vi "Init Test.vi"(10 "x":dbl, 11 "Cluster":T1) -> (3 "output cluster":T1)   [LabVIEW 2013]
uses:
  Control/SystemProcess.ctl
  Control/Buffer.vi
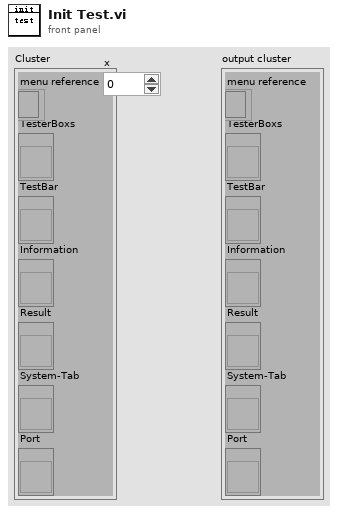
[diagram p1: front panel]
types:
  T1 = cluster{"menu reference":refnum<k9>, "TesterBoxs":refnum<vi>, "TestBar":refnum<vi>, "Information":refnum<vi>, "Result":refnum<vi>, "System-Tab":refnum<vi>, "Port":refnum<vi>}
  T2 = typedef "SystemProcess.ctl" = enum16{"Idle", "SystemInit", "SpecialEvent", "Barcode(SN)", "TestInitialize", "Test", "Stop", "SaveTestData", "Exit"}
  T3 = typedef "StatusInformation.ctl" = cluster{"FileName:":string, "Barcode(S/N):":string, "TestStep:":string, "TestTime:":string, "Station:":string, "Model:":string, "Line:":string, "Status:":string, "Series:":string, "Reserve:":string}
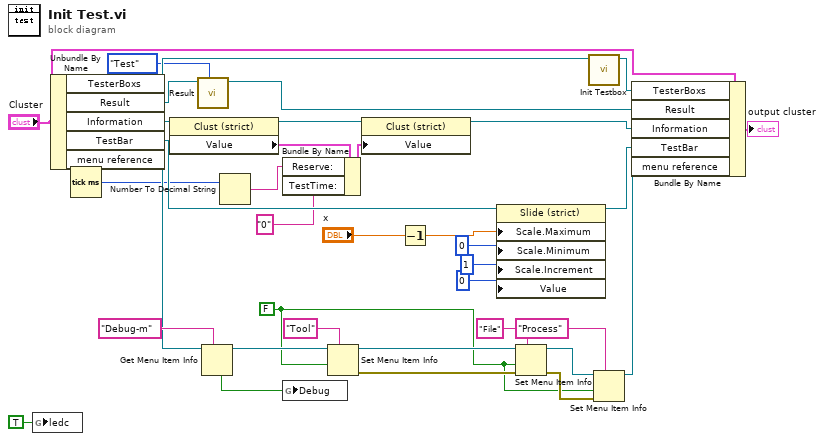
[diagram p0: block diagram]
diagram:
  w4 = FALSE ("enabled")
  n1 = global write "Buffer.vi" "ledc"(TRUE ("ledc")) -> ()
  n2 = Unbundle By Name("Cluster") -> ("TesterBoxs"=w31:refnum<vi>, "Result"=w28:refnum<vi>, "Information"=w30:refnum<vi>, "TestBar"=w33:refnum<vi>, "menu reference"=w3:refnum<k9>)
  n3 = Tick Count (ms)() -> (millisecond timer value=w1:u32)
  n4 = property class="Clust (strict)"(reference=w30) -> (reference out=w21:refnum<vi>, "Value"=w22:T3)  [unwired: 1 in, 1 out]
  n5 = call "Result.vi"("MainProcess"=SystemProcess."Test", "Result"=w28) -> ("Result"=w29:refnum<vi>)  [unwired: 9 in]
  n6 = Get Menu Item Info(7:"Debug-m" ("item tag"), 11:w3) -> (3:w17:refnum<k9>, 4:w25:bool)  [unwired: 1 in, 5 out]
  n7 = Number To Decimal String(number=w1) -> (decimal integer string=w18:string)  [unwired: 1 in]
  n8 = Bundle By Name(cluster=w22, "Reserve:"=w18, "TestTime:"="0") -> (w19:T3)
  n9 = global write "Buffer.vi" "Debug"(w25) -> ()
  n10 = Set Menu Item Info(7:"Tool" ("item tag"), 9:w4, 11:w17) -> (0:w14:errorcluster, 3:w15:refnum<k9>)  [unwired: 4 in]
  n11 = property class="Clust (strict)"(reference=w21, "Value"=w19) -> (reference out=w20:refnum<vi>)  [unwired: 1 in, 1 out]
  n12 = Decrement(x="x") -> (x-1=w23:dbl)
  n13 = property class="Slide (strict)"(reference=w33, "Scale.Maximum"=w23, "Scale.Minimum"=0 ("Data Entry Limits:Minimum"), "Scale.Increment"=1 ("Data Entry Limits:Increment"), "Value"=0) -> (reference out=w34:refnum<vi>)  [unwired: 1 in, 1 out]
  n14 = Set Menu Item Info(7:"File" ("item tag"), 8:w14, 9:w4, 11:w15) -> (0:w6:errorcluster, 3:w8:refnum<k9>)  [unwired: 3 in]
  n15 = call "Init Testbox.vi"("MulticolumnListbox in"=w31) -> ("MulticolumnListbox in"=w32:refnum<vi>)  [unwired: 10 in]
  n16 = Set Menu Item Info(7:"Process" ("item tag"), 8:w6, 9:w4, 11:w8) -> (3:w7:refnum<k9>)  [unwired: 3 in, 1 out]
  n17 = Bundle By Name(cluster="Cluster", "TesterBoxs"=w32, "Result"=w29, "Information"=w20, "TestBar"=w34, "menu reference"=w7) -> (→"output cluster":T1)
